vi "Test Process Set Self as Error Handler.vi"(8 "error in (no error)":errorcluster, 11 "Process Test In":refnum<class "Process Dev Test.lvclass">) -> (0 "error out":errorcluster, 3 "Process Test Out":refnum<class "Process Dev Test.lvclass">)   [LabVIEW 2020, in "Process Dev Test.lvclass"]
uses:
  Process Dev Test.lvclass
  C:/Program Files (x86)/National Instruments/LabVIEW 2020/vi.lib/Astemes/LUnit/Test Case.lvclass
  source/Framework/Process/Process.lvclass
  C:/Git/triarc-framework/source/Framework/Error Handler Interface/Error Handler Interface.lvclass
  source/Framework/Process/Process.lvclass/Process.ctl
  <vilib>/Astemes/LUnit/Test Case.lvclass/Test Case.ctl
  source/Framework/Process/Protected/Messaging/Send Message.vi
  source/Framework/Process/Public/Lifecycle/Get Lifecycle State.vi
  source/Framework/Process/Protected/SubVIs/Set Context.vi
  <vilib>/Utility/error.llb/Clear Errors.vi
  <vilib>/Astemes/LUnit/Add test result.vi
  <vilib>/Astemes/LUnit/Set Assertion Type.vi
  source/Framework/Process/Private/SubVIs/Handle Debug Data.vi
  source/Framework/Process/Public/Lifecycle/Leave Process Loop.vi
  <vilib>/Astemes/LUnit/LUnit Record Assertion Result.vi
  <vilib>/Utility/High Resolution Relative Seconds.vi
  <vilib>/Astemes/LUnit/LUnit Aggregate Assertion Results.vi
  <vilib>/Astemes/LUnit/Method Result/LUnit Merge Status.vi
  <vilib>/Astemes/LUnit/LUnit Concatenate result strings.vi
  <vilib>/Utility/error.llb/Error Cluster From Error Code.vi
  <vilib>/Astemes/LUnit/Test Case.lvclass
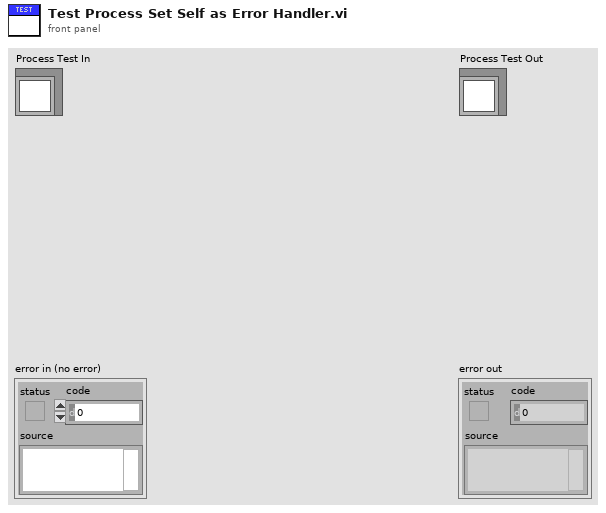
[diagram p1: front panel]
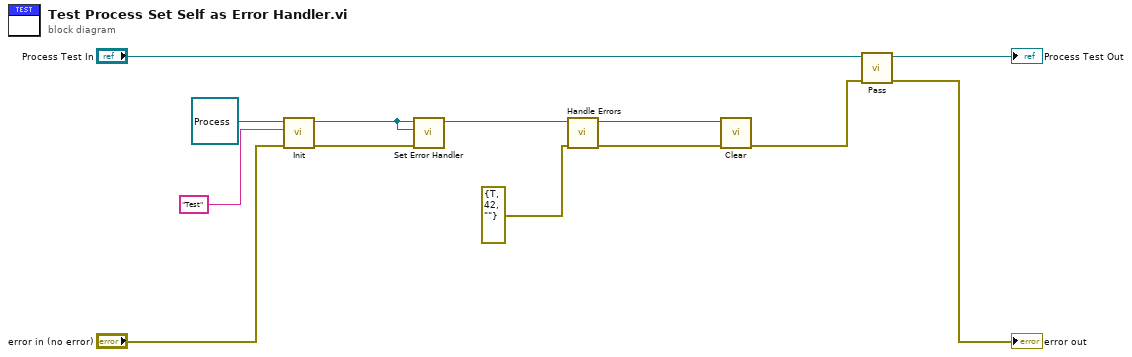
[diagram p0: block diagram]
diagram:
  n1 = call-dynamic "Init.vi"("error in (no error)"="error in (no error)", "Name"="Test", "Process In"=refnum<class "Process.lvclass"> refnum ("Process.lvclass")) -> ("error out"=w13:errorcluster, "Process Out"=w9:refnum<class "Process.lvclass">)  [unwired: 7 in]
  n2 = call "Set Error Handler.vi"("error in (no error)"=w13, "Error Handler"=w9, "Process In"=w9) -> ("Process Out"=w12:refnum<class "Process.lvclass">)  [unwired: 7 in, 1 out]
  n3 = call-dynamic "Handle Errors.vi"("error in (no error)"=errorcluster {"status"=TRUE, "code"=42, "source"=""} ("Mock Error"), "Process In"=w12) -> ("error out"=w8:errorcluster, "Process Out"=w7:refnum<class "Process.lvclass">)  [unwired: 8 in]
  n4 = call-dynamic "Clear.vi"("error in (no error)"=w8, "Process In"=w7) -> ("error out"=w6:errorcluster)  [unwired: 9 in]
  n5 = call <vilib>:"Pass.vi"("error in (no error)"=w6, "LUnit Test Case In"="Process Test In") -> ("error out"=→"error out":errorcluster, "LUnit Test Case Out"=→"Process Test Out":refnum<class "Process Dev Test.lvclass">)  [unwired: 8 in]
